vi "Display Error.vi"(1 "Cause :":string="Unknown", 3 "Source :":string="Unknown", 4 "Error? (T)":bool=TRUE) -> ()   [LabVIEW 2012]
panel:
  out "Title":string="Error Found"
  in  "OK Button":bool
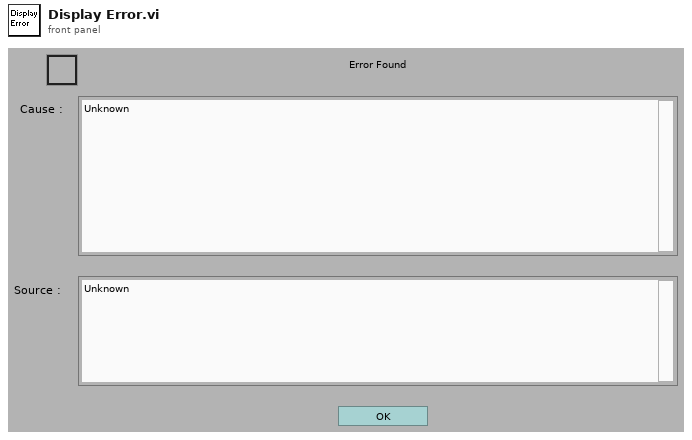
[diagram p1: front panel]
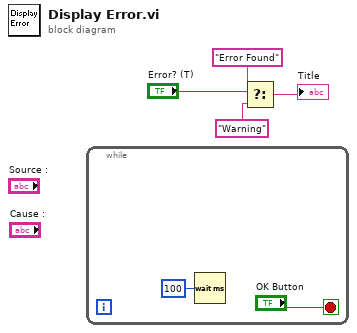
[diagram p0: block diagram]
diagram:
  n1 = while {
    stop <- "OK Button" stop-if-true
    n2 = Wait (ms)(milliseconds to wait=u32 100) -> ()  [unwired: 1 out]
  }
  n3 = Select(t="Error Found", s="Error? (T)", f="Warning") -> (s? t:f=→"Title":string)
